vi "ActionVIOnCompile.vi"(8 "error in (no error)":errorcluster, 11 "Device Item Ref in":T1 format="%.0x") -> (0 "error out":errorcluster)   [LabVIEW 2026, in "WebPage Addon System Explorer.lvlib"]
uses:
  WebPage Addon System Explorer.lvlib
  <vilib>/NI VeriStand/Custom Device API/Custom Device Item Ref.ctl
  Shared/Compiled.Settings.ctl
  <vilib>/NI VeriStand/Custom Device API/Get Item Property (Double).vi
  <vilib>/NI VeriStand/Custom Device API/Set Item Property (Variant).vi
  <vilib>/NI VeriStand/Custom Device API/Custom Device API.lvlib
  <vilib>/NI/NIVS Inline Async API/_Data Access System Explorer/Data Access System Explorer.lvlib
  Shared/WebPage Addon Shared.lvlib
  <vilib>/NI VeriStand/Custom Device API/Get Item Property (U32).vi
  <vilib>/NI VeriStand/Custom Device API/Get Item Property (String).vi
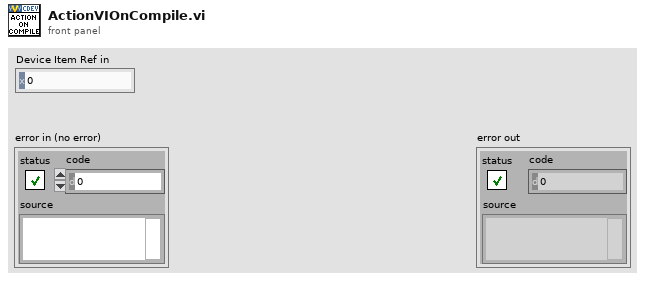
[diagram p1: front panel]
types:
  T1 = typedef "Custom Device API.lvlib/Custom Device Item Ref.ctl" = u64
  T2 = enum16{"Output/Write", "Input/Read", "Input/ReadWrite"}
  T3 = cluster{"Name":string, "Type":enum16{"Output/Write", "Input/Read", "Input/ReadWrite"}, "VS Refs":T1[]}
  T4 = typedef "WebPage Addon Shared.lvlib/Compiled.Settings.ctl" = cluster{"Name":string, "Decimation":u32, "Channel Names":string[], "Hosted IP Address":string, "Hosted Port":u32, "gRPC Port":u32}
  T5 = typedef "Custom Device API.lvlib/Custom Device Item Info.ctl" = cluster{"Name":string, "Is Channel":bool, "GUID":string, "Is Waveform":bool}
  T6 = cluster{"Name":string, "Type":enum16{"Output/Write", "Input/Read", "Input/ReadWrite"}, "VS Refs":T1[]}[]
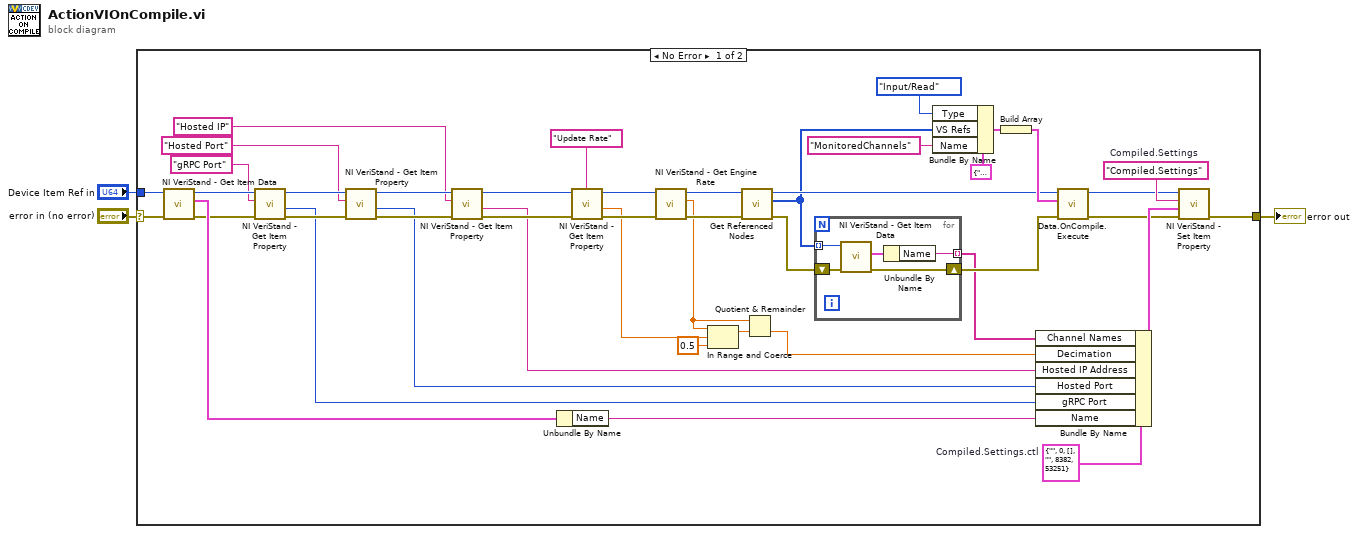
[diagram p0: block diagram]
diagram:
  n1 = case shown="No Error" "error in (no error)" {
    selector: "error in (no error)" -> [w44 w53]
    tunnel: [w45 w53] -> w2
    tunnel: "Device Item Ref in" -> [w43 _]
    frame No Error {
      w33 = T4 {"Name"="", "Decimation"=0, "Channel Names"=[], "Hosted IP Address"="", "Hosted Port"=8382, "gRPC Port"=53251}  # Compiled.Settings.ctl
      w47 = "Compiled.Settings"  # Compiled.Settings
      n2 = call <vilib>:"NI VeriStand - Get Item Data.vi"("error in (no error)"=w44, "Item Ref in"=w43) -> ("error out"=w12:errorcluster, "Item Info"=w42:T5, "Item Ref out"=w17:T1)  [unwired: 6 in, 1 out]
      n3 = call-poly <vilib>:"NI VeriStand - Get Item Property.vi"("error in (no error)"=w12, "Property Name"="gRPC Port", "Item Ref in"=w17) -> ("error out"=w11:errorcluster, "Value"=w7:u32, "Item Ref out"=w16:T1)  [unwired: 5 in, 1 out]
      n4 = call-poly <vilib>:"NI VeriStand - Get Item Property.vi"("error in (no error)"=w11, "Property Name"="Hosted Port", "Item Ref in"=w16) -> ("error out"=w10:errorcluster, "Value"=w8:u32, "Item Ref out"=w15:T1)  [unwired: 5 in, 1 out]
      n5 = call-poly <vilib>:"NI VeriStand - Get Item Property.vi"("error in (no error)"=w10, "Property Name"="Hosted IP", "Item Ref in"=w15) -> ("error out"=w13:errorcluster, "Value"=w9:string, "Item Ref out"=w14:T1)  [unwired: 5 in, 1 out]
      n6 = Unbundle By Name(w42) -> ("Name"=w41:string)
      n7 = call-poly <vilib>:"NI VeriStand - Get Item Property.vi"("error in (no error)"=w13, "Property Name"="Update Rate", "Item Ref in"=w14) -> ("error out"=w30:errorcluster, "Value"=w26:dbl, "Item Ref out"=w28:T1)  [unwired: 5 in, 1 out]
      n8 = call <vilib>:"NI VeriStand - Get Engine Rate.vi"("error in (no error)"=w30, "Item Ref in"=w28) -> ("error out"=w29:errorcluster, "Rate (Hz)"=w24:dbl, "Item Ref out"=w27:T1)  [unwired: 7 in]
      n9 = In Range and Coerce(upper limit=w24, x=w26, lower limit=0.5) -> (coerced(x)=w23:dbl)  [unwired: 1 out]
      n10 = call "Get Referenced Nodes.vi"("error in (no error)"=w29, "Item Ref in"=w27) -> ("error out"=w21:errorcluster, "Array"=w19:T1[], "Item Ref out"=w31:T1)  [unwired: 7 in]
      n11 = Quotient & Remainder(x=w24, y=w23) -> (floor(x/y)=w22:dbl)  [unwired: 1 out]
      n12 = for {
        shift-right: [w51] -> w20
        shift-left: w21 -> [w52]
        tunnel: w19 -> [w50] mode=indexing
        tunnel: [w48] -> w18 mode=indexing
        n13 = call <vilib>:"NI VeriStand - Get Item Data.vi"("error in (no error)"=w52, "Item Ref in"=w50) -> ("error out"=w51:errorcluster, "Item Info"=w49:T5)  [unwired: 6 in, 2 out]
        n14 = Unbundle By Name(w49) -> ("Name"=w48:string)
      }
      n15 = Bundle By Name(cluster=T3 {"Name"="", "Type"=enum."Output/Write", "VS Refs"=[]} ("Group"), "Type"=T2."Input/Read", "VS Refs"=w19, "Name"="MonitoredChannels" ("Item Name")) -> (w36:T3)
      n16 = Build Array(w36) -> (w38:T6)
      n17 = Bundle By Name(cluster=w33, "Channel Names"=w18, "Decimation"=w22, "Hosted IP Address"=w9, "Hosted Port"=w8, "gRPC Port"=w7, "Name"=w41) -> (w46:T4)
      n18 = call <vilib>:"Data.OnCompile.Execute.vi"("error in"=w20, "VS Ref Groups"=w38, "Custom Device Ref"=w31) -> ("error out"=w35:errorcluster, "Custom Device Ref"=w34:T1)  [unwired: 7 in]
      n19 = call-poly <vilib>:"NI VeriStand - Set Item Property.vi"("error in (no error)"=w35, "Value"=w46, "Property Name"=w47, "Item Ref in"=w34) -> ("error out"=w45:errorcluster)  [unwired: 5 in, 2 out]
    }
    frame Error {
    }
  }
  "error out" <- w2
